vi "Request Method.vi"(11 "Processing in":refnum<class "Processing.lvclass">) -> (3 "Processing out":refnum<class "Processing.lvclass">, 5 "Request Method":T1)   [LabVIEW 2020, in "HTTP Server.lvlib" / "Processing.lvclass"]
uses:
  Processing.lvclass
  lv-http-util/HTTP Utils/Request/Request.lvclass
  lv-http-util/HTTP Utils/Method.ctl
  lv-http-util/HTTP Utils/HTTP Utils.lvlib
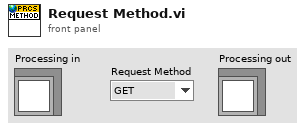
[diagram p1: front panel]
types:
  T1 = typedef "HTTP Utils.lvlib/Method.ctl" = enum16{"GET", "HEAD", "POST", "PUT", "DELETE", "CONNECT", "OPTIONS", "TRACE", "PATCH"}
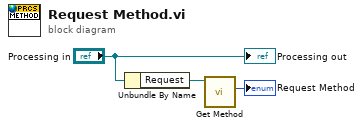
[diagram p0: block diagram]
diagram:
  n1 = Unbundle By Name("Processing in") -> ("Request"=w2:refnum<class "Request.lvclass">)
  n2 = call "Get Method.vi"("Request in"=w2) -> ("Method"=→"Request Method":T1)  [unwired: 8 in, 2 out]
  "Processing out" <- "Processing in"
